vi "Set Lower-HigherTravel Limit.vi"(4 "Travel Direction":T2, 8 "error in (no error)":errorcluster, 9 "Travel Units":T1, 10 "Limit":dbl format="%.3f", 11 "ESM303 in":refnum<class "ESM303.lvclass">) -> (0 "error out":errorcluster, 3 "ESM303 out":refnum<class "ESM303.lvclass">)   [LabVIEW 2018, in "ESM303.lvlib" / "ESM303.lvclass"]
uses:
  ESM303.lvclass
  builds/Force Test Stand/Force Test Stand/Force Test Stand.lvlibp/Custom Controls/Travel Direction.ctl
  builds/Force Test Stand/Force Test Stand/Force Test Stand.lvlibp/Custom Controls/Travel Units.ctl
  builds/Force Test Stand/Force Test Stand/Force Test Stand.lvlibp/Force Test Stand.lvclass
  C:/Projects/LabVIEW/In-Progress/Jose Rivero-Diaz/builds/Force Test Stand/Force Test Stand/Force Test Stand.lvlibp/Force Test Stand.lvclass
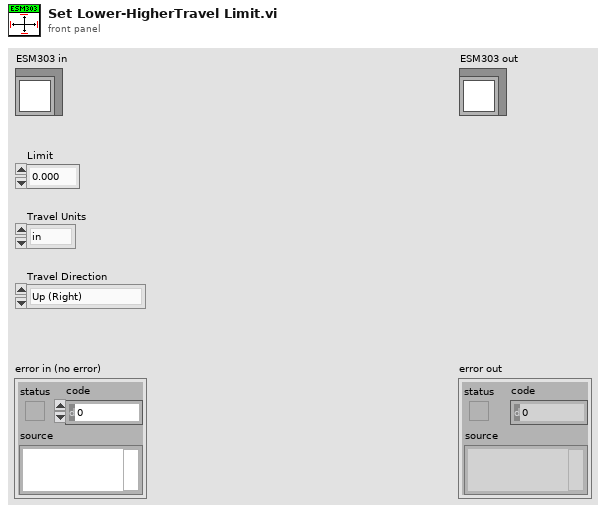
[diagram p1: front panel]
types:
  T1 = typedef "Force Test Stand.lvlibp/Force Test Stand.lvclass/Travel Units.ctl" = enum16{"in", "mm"}
  T2 = typedef "Force Test Stand.lvlibp/Force Test Stand.lvclass/Travel Direction.ctl" = enum16{"Up (Right)", "Down (Left)"}
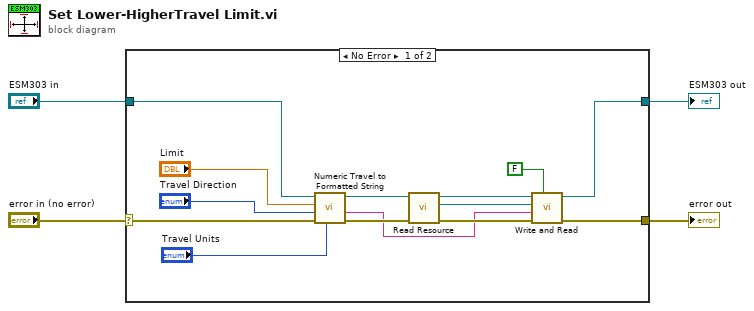
[diagram p0: block diagram]
diagram:
  n1 = case shown="No Error" "error in (no error)" {
    selector: "error in (no error)" -> [w16 w20]
    tunnel: [w5 w20] -> w3
    tunnel: [w6 w19] -> w2
    tunnel: "ESM303 in" -> [w7 w19]
    frame No Error {
      n2 = call "Numeric Travel to Formatted String.vi"("Travel Units"="Travel Units", "error in (no error)"=w16, "Travel Direction"="Travel Direction", "Travel"="Limit", "ESM303 in"=w7) -> ("error out"=w13:errorcluster, "Formatted Travel String"=w8:string, "ESM303 out"=w14:refnum<class "ESM303.lvclass">)  [unwired: 4 in]
      n3 = call "Read Resource.vi"("error in (no error)"=w13, "Force Test Stand in"=w14) -> ("error out"=w11:errorcluster, "Resource"=w10:refnum<visa-resource-name>, "Force Test Stand out"=w12:refnum<class "ESM303.lvclass">)  [unwired: 7 in]
      n4 = call "Write and Read.vi"("Write & Read"=FALSE, "error in (no error)"=w11, "Command"=w8, "VISA Refnum in"=w10, "ESM303 in"=w12) -> ("error out"=w5:errorcluster, "ESM303 out"=w6:refnum<class "ESM303.lvclass">)  [unwired: 4 in, 1 out]
    }
    frame Error {
    }
  }
  "error out" <- w3
  "ESM303 out" <- w2
